vi "Example-I2C.vi"() -> ()   [LabVIEW 2018]
panel:
  in  "Frequency(Hz)":i32(ring)=400 items=["1"=1, "10"=10, "40"=40, "100"=100, "400"=400, "1000"=1000, "4000"=4000, "10000"=10000, "40000"=40000, "100000"=100000, "400000"=400000, "1000000"=1000000, "4000000"=4000000, "10000000"=10000000]
  in  "RxLen":i32=3
  in  "addr":u8=96 format="%.0x"
  out "数值":i32
  out "波形图":u8[](graph)
  out "SerialNumber":string
  out "rxcount out":i32
  out "rgRX":u8[](array[numeric])
  in  "Tx data":u8[](array[numeric])
  in  "SDA IO(0~15)":i32=1
  in  "SCL IO(0~15)":i32
  out "returns":i32[](array[numeric])
  out "error out":errorcluster caption="错误输出"
  in  "error in (no error)":errorcluster caption="错误输入（无错误）"
  out "ftHandle out":u64=363562184
  in  "设备索引":i32
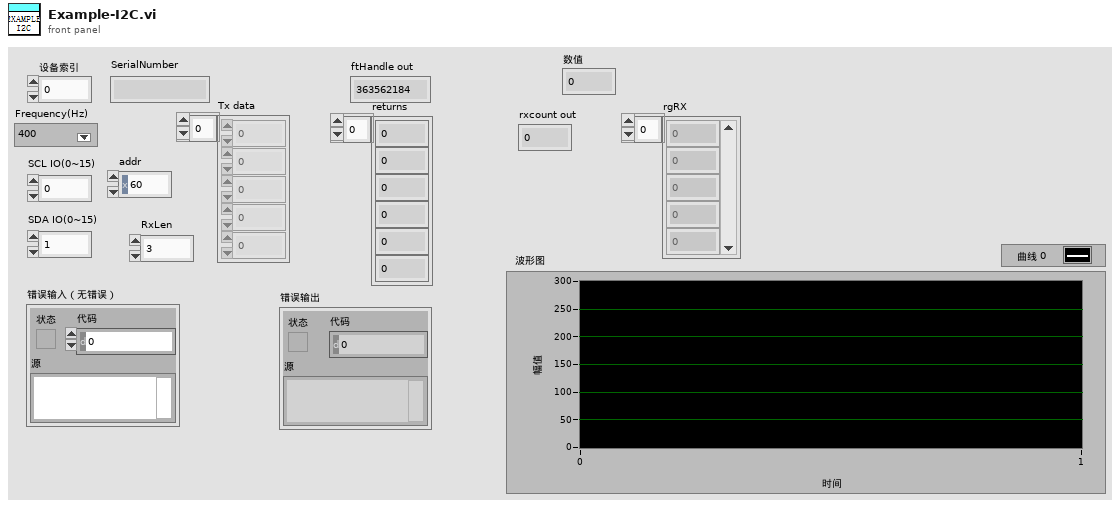
[diagram p1: front panel]
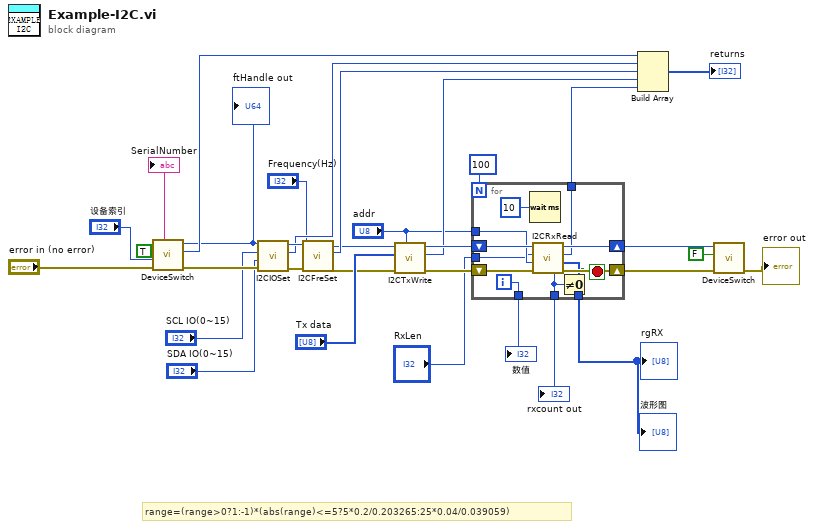
[diagram p0: block diagram]
diagram:
  # "range=(range>0?1:-1)*(abs(range)<=5?5*0.2/0.203265:25*0.04/0.039059)"
  n1 = call "DeviceSwitch.vi"("error in (no error)"="error in (no error)", "Device Index"="设备索引", "Open"=TRUE) -> ("error out"=w25:errorcluster, "function return"=w28:i32, "handle out"=w8:u64, "SerialNumber"=→"SerialNumber":string)  [unwired: 4 in, 1 out]
  "ftHandle out" <- w8
  n2 = call "I2CIOSet.vi"("error in (no error)"=w25, "SDA IO(0~15)"="SDA IO(0~15)", "SCL IO(0~15)"="SCL IO(0~15)", "handle"=w8) -> ("error out"=w24:errorcluster, "function return"=w20:i32, "handle out"=w21:u64)  [unwired: 5 in]
  n3 = call "I2CFreSet.vi"("error in (no error)"=w24, "Frequency(Hz)"="Frequency(Hz)", "handle"=w21) -> ("error out"=w15:errorcluster, "function return"=w19:i32, "handle out"=w18:u64)  [unwired: 6 in]
  n4 = call "I2CTxWrite.vi"("addr"="addr", "error in (no error)"=w15, "data"="Tx data", "handle"=w18) -> ("error out"=w16:errorcluster, "function return"=w11:i32, "handle out"=w12:u64)  [unwired: 5 in]
  n5 = for {
    N: 100 -> [_]
    tunnel: [w40] -> w10
    tunnel: [w39] -> w5
    tunnel: [w38] -> w7
    shift-right: [w43] -> w14
    shift-left: w16 -> [w44]
    shift-right: [w42] -> w13
    shift-left: w12 -> [w41]
    tunnel: [w35] -> w4
    tunnel: "addr" -> [w34]
    tunnel: "RxLen" -> [w33]
    i -> [w35]
    stop <- w37 stop-if-true
    n6 = Wait (ms)(milliseconds to wait=u32 10 ("等待时间（毫秒）")) -> ()  [unwired: 1 out]
    n7 = call "I2CRxRead.vi"("error in (no error)"=w44, "addr"=w34, "length"=w33, "handle"=w41) -> ("error out"=w43:errorcluster, "rgRX"=w39:u8[], "function return"=w40:i32, "handle out"=w42:u64, "rxcount out"=w38:i32)  [unwired: 3 in]
    n8 = Not Equal To 0?(x=w38) -> (x != 0?=w37:bool)
  }
  "rgRX" <- w5
  "rxcount out" <- w7
  "波形图" <- w5
  "数值" <- w4
  n9 = Build Array(w28, w20, w19, w11, w10) -> (→"returns":i32[])
  n10 = call "DeviceSwitch.vi"("error in (no error)"=w14, "Open"=FALSE, "handle"=w13) -> ("error out"=→"error out":errorcluster)  [unwired: 4 in, 4 out]
